vi "setStrain.vi"(6 "Channel":i32, 8 "error in (no error)":errorcluster, 9 "Slew (V/s)":dbl, 10 "Strain (V)":dbl, 11 "Instrument.Strain in":refnum<class "Instrument.Strain.lvclass">) -> (0 "error out":errorcluster, 3 "Instrument.Strain out":refnum<class "Instrument.Strain.lvclass">)   [LabVIEW 2019, in "Instrument.Strain.lvclass"]
uses:
  Instrument.Strain.lvclass
  C:/Users/patrick/Documents/GitHub/Instrument-Framework/lvsrc/Instrument/Instrument.lvclass
  Typedefs/setStrain--cluster.ctl
  daf8fb51-d54f-42e3-8e45-465e7be1bd22.vi
  daf8fb51-d54f-42e3-8e45-465e7be1bd22.vi/449805a5-d325-490e-a58a-58416a3832ef.vi
  daf8fb51-d54f-42e3-8e45-465e7be1bd22.vi/449805a5-d325-490e-a58a-58416a3832ef.vi/795b5e2a-814f-4604-ab58-6dc908b72963.vi
  daf8fb51-d54f-42e3-8e45-465e7be1bd22.vi/449805a5-d325-490e-a58a-58416a3832ef.vi/fab6e76d-9848-41af-91e0-1e51cddeede8.vi
  Instrument/Private/Get RC Connection Status.vi
  Instrument/API/Send and Receive.vi
  <vilib>/Utility/Data Type/Get Type Information.vi
  <vilib>/JDP Science/JSONtext/JSON text to Variant.vi
  <vilib>/JDP Science/JSONtext/LVClass Serializer/JSONtext LVClass Serializer.lvclass
  Instrument/Instrument.lvclass
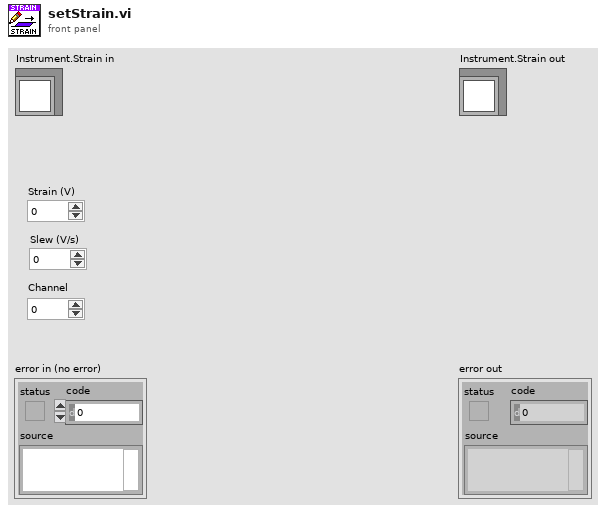
[diagram p1: front panel]
types:
  T1 = typedef "Instrument.Strain.lvclass/setStrain--cluster.ctl" = cluster{"strain":dbl, "slew":dbl, "channel":i32}
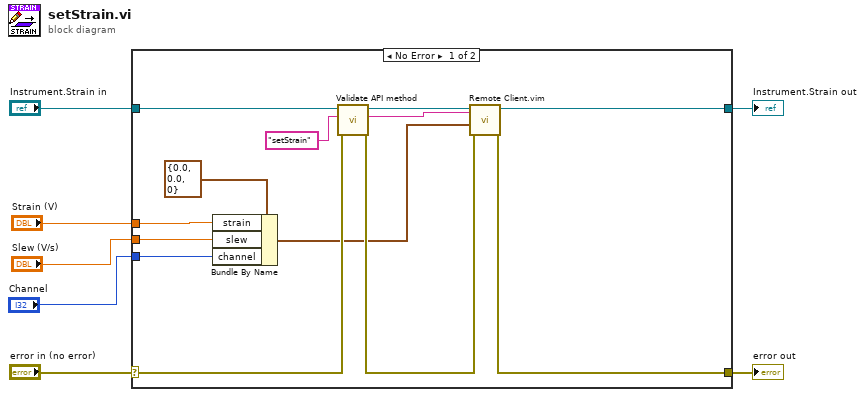
[diagram p0: block diagram]
diagram:
  n1 = case shown="No Error" "error in (no error)" {
    selector: "error in (no error)" -> [w15 w22]
    tunnel: [w13 w22] -> w6
    tunnel: [w16 w21] -> w4
    tunnel: "Instrument.Strain in" -> [w17 w21]
    tunnel: "Strain (V)" -> [w11 _]
    tunnel: "Slew (V/s)" -> [w10 _]
    tunnel: "Channel" -> [w9 _]
    frame No Error {
      n2 = Bundle By Name(cluster=T1 {"strain"=0.0, "slew"=0.0, "channel"=0} ("setStrain"), "strain"=w11, "slew"=w10, "channel"=w9) -> (w8:T1)
      n3 = call "Validate API method.vi"("error in (no error)"=w15, "Command in"="setStrain" ("error message (\"\")"), "Instrument in"=w17) -> ("error out"=w14:errorcluster, "command out"=w19:string, "Instrument out"=w18:refnum<class "Instrument.Strain.lvclass">)  [unwired: 6 in]
      n4 = call "Remote Client.vim"("Data Out type"=w19, "error in (no error)"=w14, "Data in"=w8, "Instrument in"=w18) -> ("error out"=w13:errorcluster, "Instrument out"=w16:refnum<class "Instrument.Strain.lvclass">)  [unwired: 4 in, 2 out]
    }
    frame Error {
    }
  }
  "error out" <- w6
  "Instrument.Strain out" <- w4
